vi "Transducer Selection.vi"(7 "error in (no error)":errorcluster, 10 "Connection Data In":T1) -> (0 "error out":errorcluster, 1 "Range":dbl, 2 "Index":u64, 3 "Connection Data Out":T1)   [LabVIEW 2014, in "MSX-E3701_dll.lvlib"]
doc: "Adquiere la información que leyó el VI de TransducerTypeInformation y permite al usuario elegir el transductor que se va a medir."
uses:
  MSX-E3701_dll.lvlib
  Typedef/Calibration Data.ctl
  Typedef/Connection Data.ctl
  E:/Repositorio Magnis/INF002/v0/Modules/HAL/Drivers/Sync/ADDI-DATA MSX-E3701/API/MX370x.dll
  MX370x.dll
  E:/Repositorio Magnis/INF002/v0/Modules/HAL/Drivers/Sync/ADDI-DATA MSX-E3701/API/MXCommon.dll
  MXCommon.dll
panel:
  in  "View Transducers":bool=TRUE
  in  "Add Transducer":bool=TRUE
  out "Cluster Calibration":T2
  # "Transducer Selection"
  # "Information"
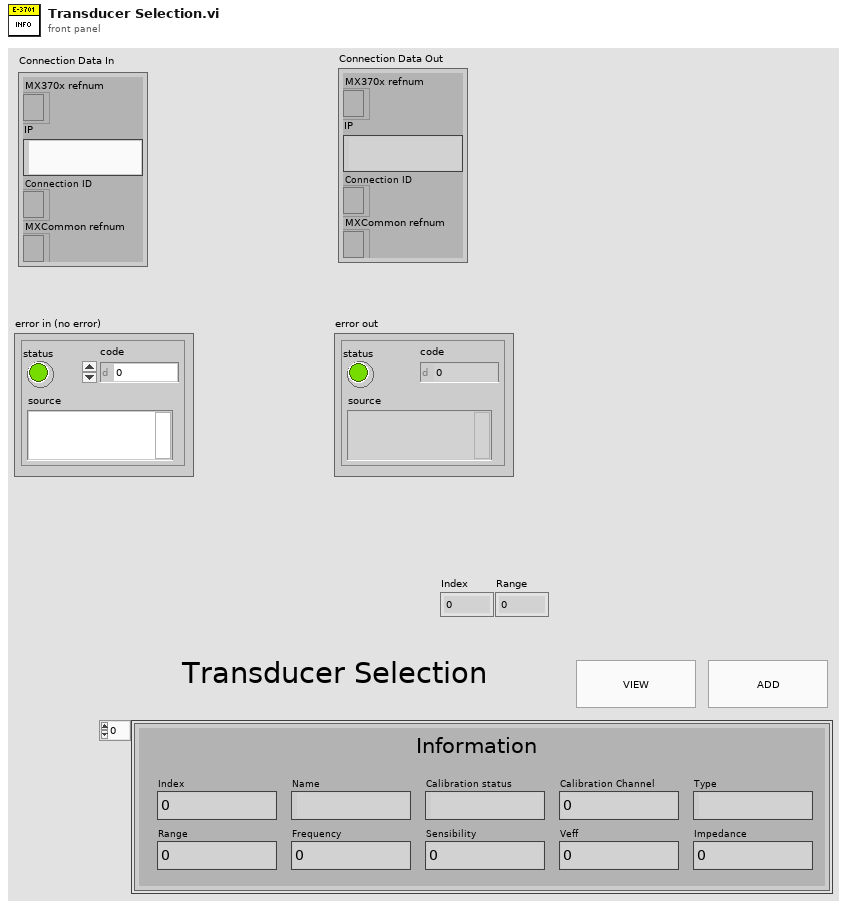
[diagram p1: front panel]
types:
  T1 = typedef "MSX-E3701_dll.lvlib/Connection Data.ctl" = cluster{"MX370x refnum":refnum<k24>, "IP":string, "Connection ID ":refnum<k5>, "MXCommon refnum":refnum<k24>}
  T2 = typedef "MSX-E3701_dll.lvlib/Calibration Data.ctl" = cluster{"Calibration status":string, "Name":string, "Index":u64, "Range":dbl, "Sensibility":dbl, "Veff":dbl, "Frequency":u64, "Impedance":u64, "Type":string, "Calibration Channel":u64}[]
  T3 = cluster{"Calibration status":string, "Name":string, "Index":u64, "Range":dbl, "Sensibility":dbl, "Veff":dbl, "Frequency":u64, "Impedance":u64, "Type":string, "Calibration Channel":u64}
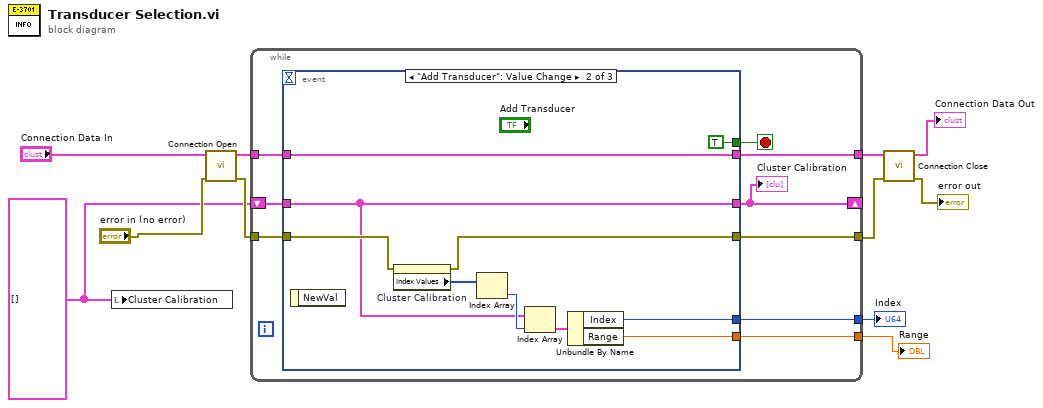
[diagram p0: block diagram]
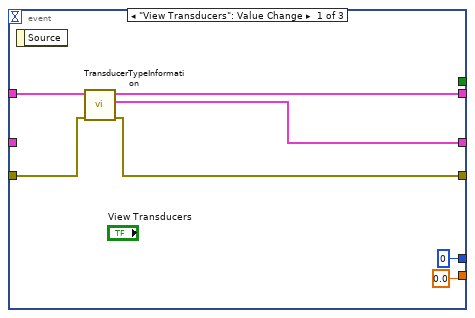
[diagram p2: hidden frame]
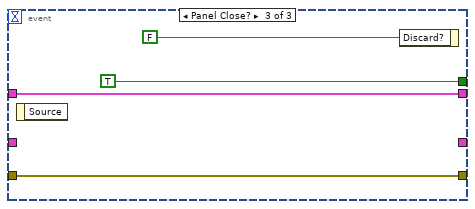
[diagram p3: hidden frame]
diagram:
  w2 = T2 [] ("Cluster Calibration")
  n1 = local write "Cluster Calibration"(w2) -> ()
  n2 = call "Connection Open.vi"("Error In"="error in (no error)", "Connection Data In"="Connection Data In") -> ("Error Out"=w6:errorcluster, "Connection Data Out"=w7:T1)  [unwired: 8 in]
  n3 = while {
    tunnel: w7 -> [w19]
    tunnel: w6 -> [w18]
    tunnel: [w17] -> w10
    tunnel: [w16] -> w9
    shift-right: [w14] -> _
    shift-left: w2 -> [w15]
    tunnel: [w13] -> w1
    tunnel: [w12] -> w3
    stop <- w20 stop-if-true
    n4 = event shown="[1] \"Add Transducer\": Value Change" {
      selector: _ -> [_ _ _]
      dyn-events: _ -> [_ _ _]
      timeout: _ -> [_ _ _]
      tunnel: [_ TRUE ("Discard?") TRUE ("Discard?")] -> w20
      tunnel: w19 -> [w27 w37 w39]
      tunnel: w18 -> [w26 w33 w38]
      tunnel: [w25 w37 w39] -> w17
      tunnel: [w24 w32 w38] -> w16
      tunnel: [w23 w29 _] -> w14
      tunnel: w15 -> [_ w29 _]
      tunnel: [0.0 ("Range") w31 _] -> w13
      tunnel: [u64 0 ("Index") w30 _] -> w12
      event "View Transducers": Value Change {
        n5 = event-data() -> ()  [unwired: 1 in, 1 out]
        n6 = call "TransducerTypeInformation.vi"("error in (no error)"=w26, "Connection Data In"=w27) -> ("error out"=w24:errorcluster, "Cluster Calibration"=w23:T2, "Connection Data Out"=w25:T1)  [unwired: 7 in]
      }
      event "Add Transducer": Value Change {
        n7 = event-data() -> ()  [unwired: 1 in, 1 out]
        n8 = property on="Cluster Calibration" class="Arr (strict)"(error in=w33) -> (error out=w32:errorcluster, "Index Values"=w34:u32[])  [unwired: 1 in, 1 out]
        n9 = Index Array(array=w34) -> (element=w36:u32)  [unwired: 1 in]
        n10 = Index Array(array=w29, index=w36) -> (element=w35:T3)
        n11 = Unbundle By Name(w35) -> ("Index"=w30:u64, "Range"=w31:dbl)
      }
      event Panel Close? {
        n12 = event-data() -> ()  [unwired: 1 in, 1 out]
        n13 = event-data("Discard?"=FALSE) -> ()  [unwired: 1 in, 1 out]
      }
    }
    "Cluster Calibration" <- w14
  }
  "Index" <- w3
  "Range" <- w1
  n14 = call "Connection Close.vi"("error in (no error)"=w9, "Connection Data In"=w10) -> ("error out"=→"error out":errorcluster, "Connection Data Out"=→"Connection Data Out":T1)  [unwired: 8 in]
